vi "Match_CMC.vi"(6 "CMC IN":string[][](array[string]), 8 "error in":errorcluster caption="에러 입력(에러 없음)", 9 "Condition IN":string[][](array[string]), 11 "Func_ext":string) -> (0 "error out":errorcluster caption="에러 출력", 1 "에러?":bool, 2 "CMC Out":string[][](array[string]), 3 "Func_ext out":string)   [LabVIEW 2020]
uses:
  Controls/Cmd_Var Data IO.ctl
panel:
  # "0, DSEQ\n1, CLSMAN\n2, CLSMAN_EXT\n3, FUNC\n4, FUNC_EXT\n5, FUNC_CON\n6, C1_LOW\n7, C1_LUNIT\n8, C1_LCON\n9, C1_HIGH\n10, C1_HUNIT\n11, C1_HCON\n12, RANGE_LOW\n13, RANGE_LUNIT\n14, RANGE_LDIV\n15, RANGE_HIGH\n16, RANGE_HUNIT\n17, RANGE_HDIV\n18, CMC1_VAL\n19, CMC2_VAL\n20, CMC_UNIT"
  # "0, FUNC\n1, FUNC_EXT\n2, FUNC_CON\n3, C1_VAL\n4, C1_UNIT\n5, RANGE_VAL\n6, RANGE_UNIT"
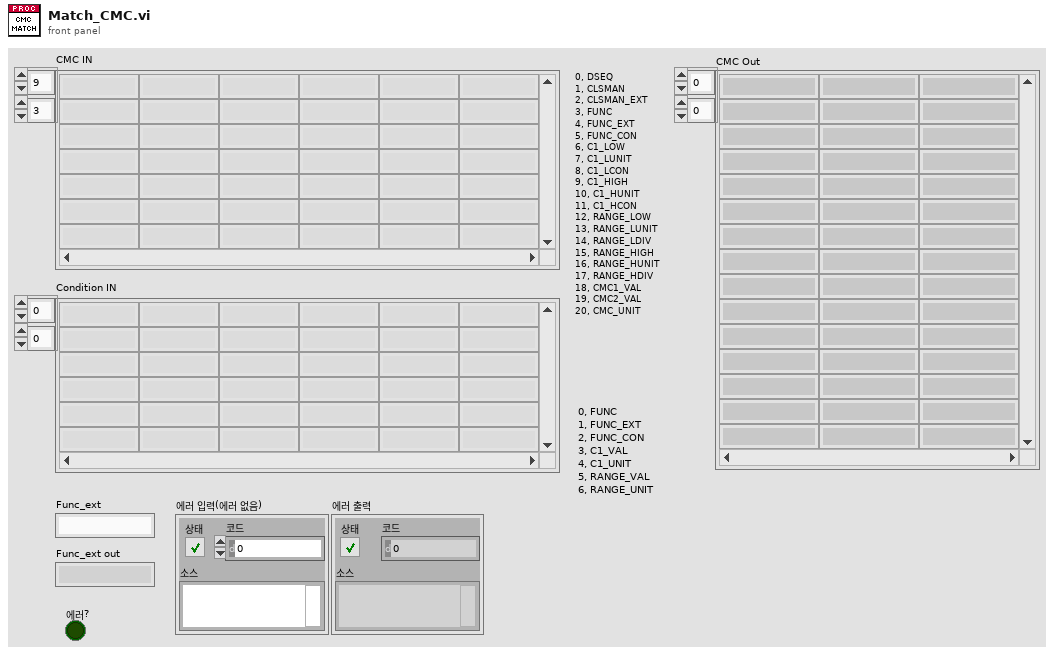
[diagram p1: front panel]
types:
  T1 = typedef "Cmd_Var Data IO.ctl" = enum16{"Condition", "Condition Default", "Condition_Temp", "Resolution", "Resolution Default", "Resolution Old", "Spec", "Spec Default", "Spec Old", "Spec Temp", "Result", "Result2", "Result3", "Result_Temp", "Result_ADJ", "Result_ADJ2", "STD1", "STD2", "STD3", "STD4", "STD5", "STD Temp", "CMC", "CMC Default"}
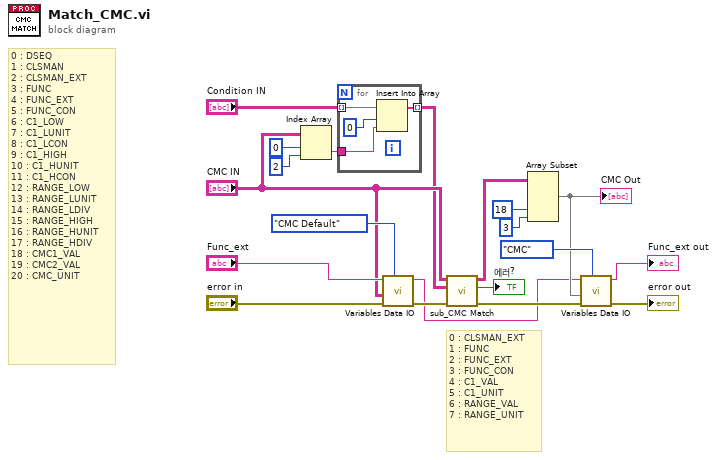
[diagram p0: block diagram]
diagram:
  # "0 : CLSMAN_EXT\n1 : FUNC\n2 : FUNC_EXT\n3 : FUNC_CON\n4 : C1_VAL\n5 : C1_UNIT\n6 : RANGE_VAL\n7 : RANGE_UNIT"
  # "0 : DSEQ\n1 : CLSMAN\n2 : CLSMAN_EXT\n3 : FUNC\n4 : FUNC_EXT\n5 : FUNC_CON\n6 : C1_LOW\n7 : C1_LUNIT\n8 : C1_LCON\n9 : C1_HIGH\n10 : C1_HUNIT\n11 : C1_HCON\n12 : RANGE_LOW\n13 : RANGE_LUNIT\n14 : RANGE_LDIV\n15 : RANGE_HIGH\n16 : RANGE_HUNIT\n17 : RANGE_HDIV\n18 : CMC1_VAL\n19 : CMC2_VAL\n20 : CMC_UNIT"
  n1 = Index Array(array="CMC IN", index (row)=0 ("비활성화된 인덱스 (행)"), index (col)=2 ("비활성화된 인덱스 (열)")) -> (element=w11:string)
  n2 = for {
    tunnel: w11 -> [w23]
    tunnel: [w22] -> w2 mode=indexing
    tunnel: "Condition IN" -> [w21] mode=indexing
    n3 = Insert Into Array(array=w21, index=0 ("인덱스"), new element=w23) -> (w22:string[])
  }
  n4 = call "Variables Data IO.vi"("Select"=Cmd_Var_Data_IO."CMC Default", "Data In"="CMC IN", "Func_ext"="Func_ext") -> ("Func_ext Out"=w5:string)  [unwired: 6 in, 2 out]
  n5 = call "sub_CMC Match.vi"("error in (no error)"="error in", "DATA IN"=w2, "CMC IN"="CMC IN") -> ("error out"=w9:errorcluster, "에러?"=→"에러?":bool, "CMC Out"=w8:string[][])  [unwired: 6 in]
  n6 = Array Subset(array=w8, index (col)=18 ("인덱스"), length (col)=3 ("길이")) -> (w15:string[][])  [unwired: 2 in]
  "CMC Out" <- w15
  n7 = call "Variables Data IO.vi"("Select"=Cmd_Var_Data_IO."CMC", "error in"=w9, "Data In"=w15, "Func_ext"=w5) -> ("error out"=→"error out":errorcluster, "Func_ext Out"=→"Func_ext out":string)  [unwired: 5 in, 1 out]
